vi "CH1_Tx.vi"() -> ()   [LabVIEW 2018]
uses:
  RxTx/RxTx.lvclass
  Stream/Stream.lvclass
panel:
  in  "RxTx.lvclass":refnum<class "RxTx.lvclass">
  in  "Stream.lvclass":refnum<class "Stream.lvclass">
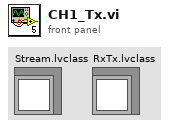
[diagram p1: front panel]
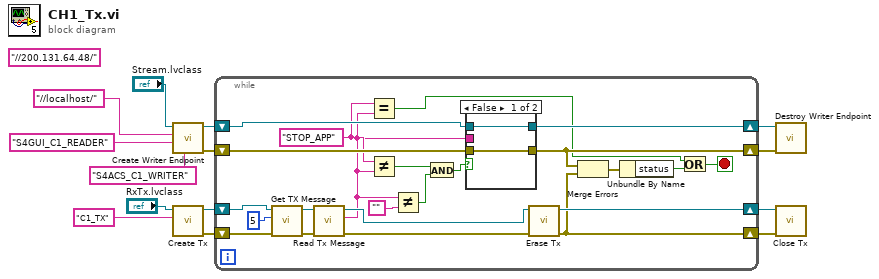
[diagram p0: block diagram]
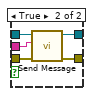
[diagram p2: hidden frame]
diagram:
  (unwired) "//200.131.64.48/" ("Reader Name")
  n1 = call "Create Writer Endpoint.vi"("writer name"="S4ACS_C1_WRITER" ("reader name"), "reader name"="S4GUI_C1_READER", "IP"="//localhost/" ("Reader Name"), "Stream in"="Stream.lvclass") -> ("error out"=w5:errorcluster, "Stream out"=w7:refnum<class "Stream.lvclass">)  [unwired: 6 in]
  n2 = call "Create Tx.vi"("Writer Name"="C1_TX" ("Reader Name"), "RxTx in"="RxTx.lvclass") -> ("error out"=w12:errorcluster, "RxTx out"=w13:refnum<class "RxTx.lvclass">)  [unwired: 8 in]
  n3 = while {
    shift-right: [w28] -> w3
    shift-left: w5 -> [w30]
    shift-right: [w29] -> w14
    shift-left: w7 -> [w31]
    shift-right: [w23] -> w8
    shift-left: w12 -> [w32]
    shift-right: [w25] -> w9
    shift-left: w13 -> [w33]
    stop <- w20 stop-if-true
    w19 = "STOP_APP"
    n4 = call "Get TX Message.vi"("error in (no error)"=w32, 10:5 ("timeout in ms"), "RxTx in"=w33) -> ("error out"=w36:errorcluster, "RxTx out"=w35:refnum<class "RxTx.lvclass">)  [unwired: 7 in]
    n5 = call "Read Tx Message.vi"("error in (no error)"=w36, "RxTx in"=w35) -> ("error out"=w24:errorcluster, "Tx Message"=w18:string, "RxTx out"=w26:refnum<class "RxTx.lvclass">)  [unwired: 7 in]
    n6 = Equal?(x=w19, y=w18) -> (x = y?=w22:bool)
    n7 = Not Equal?(x=w19, y=w18) -> (x != y?=w17:bool)
    n8 = Not Equal?(x=w18, y="") -> (x != y?=w16:bool)
    n9 = And(x=w17, y=w16) -> (x .and. y?=w15:bool)
    n10 = case shown="False" w15 {
      tunnel: w31 -> [w39 w44]
      tunnel: w30 -> [w38 w43]
      tunnel: [w39 w42] -> w29
      tunnel: w18 -> [_ w41]
      tunnel: [w38 w40] -> w28
      frame False {
      }
      frame True {
        n11 = call "Send Message.vi"("error in (no error)"=w43, "Message"=w41, "Stream in"=w44) -> ("error out"=w40:errorcluster, "Stream out"=w42:refnum<class "Stream.lvclass">)  [unwired: 7 in]
      }
    }
    n12 = call "Erase Tx.vi"("error in (no error)"=w24, "RxTx in"=w26) -> ("error out"=w23:errorcluster, "RxTx out"=w25:refnum<class "RxTx.lvclass">)  [unwired: 8 in]
    n13 = Merge Errors(w28, w23) -> (w37:errorcluster)
    n14 = Unbundle By Name(w37) -> ("status"=w21:bool)
    n15 = Or(x=w22, y=w21) -> (x .or. y?=w20:bool)
  }
  n16 = call "Destroy Writer Endpoint.vi"("error in (no error)"=w3, "Stream in"=w14) -> ()  [unwired: 8 in, 2 out]
  n17 = call "Close Tx.vi"("error in (no error)"=w8, "RxTx in"=w9) -> ()  [unwired: 8 in, 2 out]
